vi "Micro-Epsilon ILD1420.vi"() -> (0 "DAQ Error":errorcluster)   [LabVIEW 2016]
uses:
  Globals/Meas_global.vi
panel:
  out "Waveform Graph":cluster{"y":dbl, dbl, "d (mm)":dbl[]}(graph)
  in  "Reconfigure settings":bool
  in  "Data rate (kHz)":string(combo)="0.25"
  in  "Measuring range (mm)":u8(ring)=4 items=["10", "25", "50", "100", "200"]
  in  "Auto laser off":bool=TRUE
  # "(set true if changing data rate)"
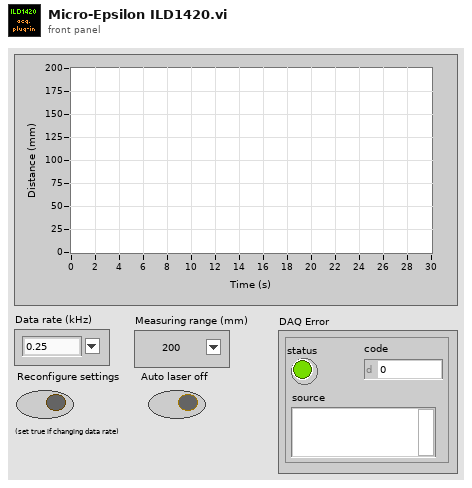
[diagram p1: front panel]
types:
  T1 = typedef "Analysis_info_cluster.ctl" = cluster{"Colour":u32, "Inst type":T2, "Inst name":string, "Symbol":string, "Code name":string, "Extra Info":string, "Inst Array":T3, "Extra Titles":string[], "Extra Values":string[], "U":dbl, "u^2":dbl, "u^3":dbl, "u^4":dbl, "Skew_u":dbl, "Kurt_u":dbl, "Sd Error in Mean":dbl, "% u'/U":dbl, "X":dbl, "Y":dbl, "Z":dbl, "Timescale integral Estimate":dbl, "Sd Error in Variance":dbl, "Calib File":path, "Calib Constants":dbl[], "Output Position":bool, "Full Stats":bool, "Av Sampling Rate":dbl, "Av No of Samples":dbl, "Total Meas Time (s)":dbl, "ADAM Ch Name":string, "Max value":dbl, "Min value":dbl}
  T2 = typedef "Inst_type.ctl" = enum16{"Propeller anemometer", "Raw voltage", "Pressure Transducer", "Pitot-static tube", "Preston tube", "Hot wire", "Cross wire 1", "Cross wire 2", "Generic Linear", "Generic Polynomial", "Generic BackPoly", "Fast FID", "Thermocouple", "Cold wire", "Pulsed Wire", "LDA Vel", "LDA Tran time", "LDA Arr time", "Microphone"}
  T3 = typedef "Instrument_Array.ctl" = enum16{"PWA", "LDA", "Analogue"}
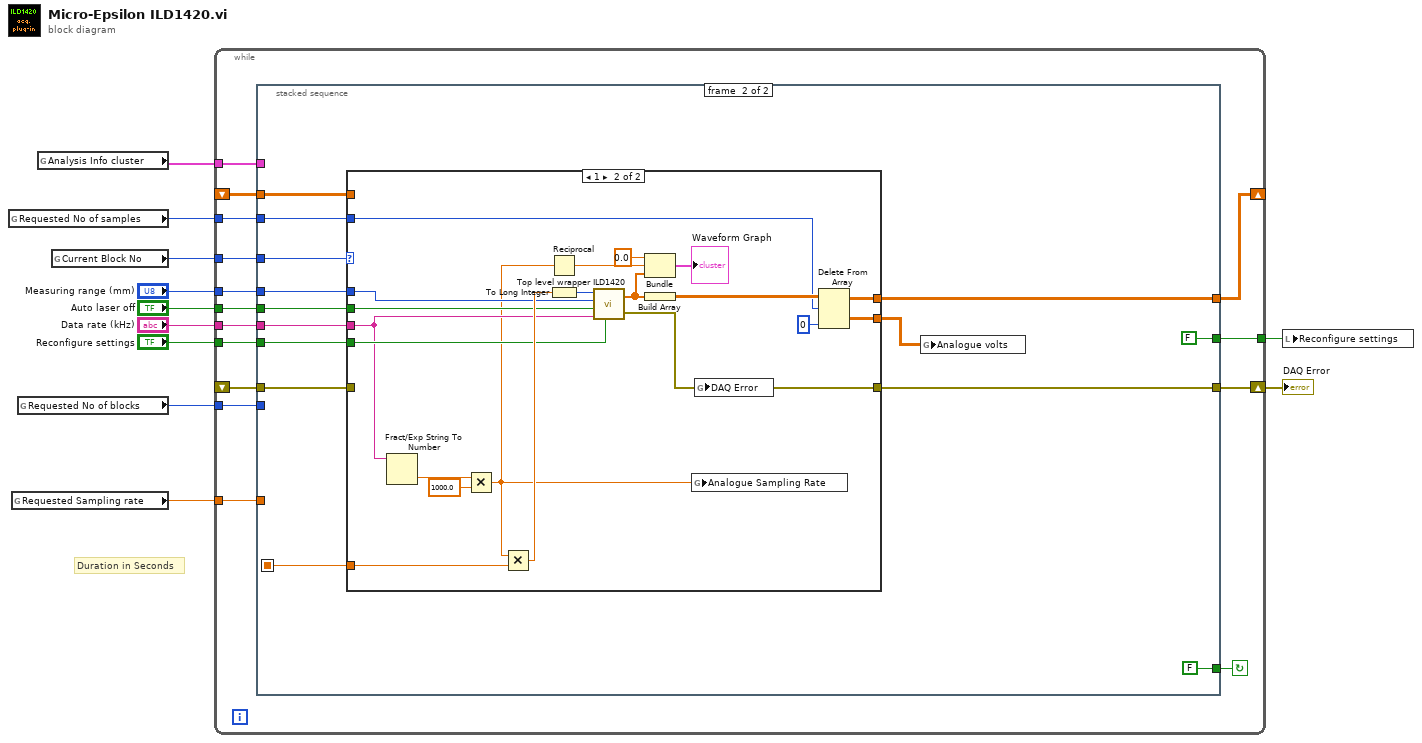
[diagram p0: block diagram]
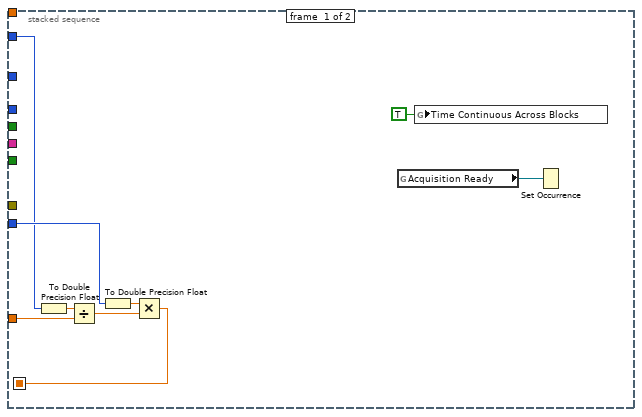
[diagram p2: hidden frame]
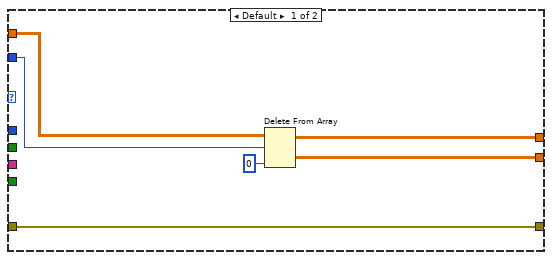
[diagram p3: hidden frame]
diagram:
  # "Duration in Seconds"
  n1 = global read "Meas_global.vi" "Requested No of samples"() -> (w11:i32)
  n2 = global read "Meas_global.vi" "Requested Sampling rate"() -> (w10:dbl)
  n3 = global read "Meas_global.vi" "Requested No of blocks"() -> (w7:i32)
  n4 = global read "Meas_global.vi" "Analysis Info cluster"() -> (w8:T1[])
  n5 = global read "Meas_global.vi" "Current Block No"() -> (w9:i32)
  n6 = while {
    tunnel: w11 -> [w26]
    tunnel: w10 -> [w25]
    tunnel: w9 -> [w24]
    tunnel: w8 -> [w23]
    tunnel: w7 -> [w22]
    tunnel: "Measuring range (mm)" -> [w20]
    tunnel: "Auto laser off" -> [w19]
    tunnel: "Data rate (kHz)" -> [w18]
    shift-right: [w14] -> _
    shift-left: _ -> [w12]
    tunnel: "Reconfigure settings" -> [w17]
    tunnel: [w16] -> w1
    shift-right: [w21] -> w6
    shift-left: _ -> [w13]
    stop <- w15 continue-if-true
    n7 = stacked-sequence {
      seq-local: [w32 _] -> [_ w49]
      tunnel: w26 -> [w31 w40]
      tunnel: w24 -> [_ w42]
      tunnel: w23 -> [_ _]
      tunnel: w25 -> [w35 _]
      tunnel: w22 -> [w33 _]
      tunnel: [_ w48] -> w21
      tunnel: w20 -> [_ w47]
      tunnel: w19 -> [_ w46]
      tunnel: w18 -> [_ w44]
      tunnel: w17 -> [_ w45]
      tunnel: [_ FALSE ("Reconfigure settings")] -> w16
      tunnel: [_ FALSE ("Reconfigure settings")] -> w15
      tunnel: [_ w39] -> w14
      tunnel: w13 -> [_ w38]
      tunnel: w12 -> [_ w37]
      frame #0 {
        n8 = To Double Precision Float(number=w31) -> (double precision float=w28:dbl)
        n9 = Divide(x=w28, y=w35) -> (x/y=w34:dbl)
        n10 = To Double Precision Float(number=w33) -> (double precision float=w27:dbl)
        n11 = Multiply(x=w27, y=w34) -> (x*y=w32:dbl)
        n12 = global read "Meas_global.vi" "Acquisition Ready"() -> (w29:refnum<k4>)
        n13 = global write "Meas_global.vi" "Time Continuous Across Blocks"(TRUE ("Time Continuous across Blocks")) -> ()
        n14 = Set Occurrence(w29) -> ()
      }
      frame #1 {
        n15 = case shown="1" w42 {
          tunnel: w49 -> [_ w75]
          tunnel: [w55 w73] -> w48
          tunnel: w47 -> [_ w71]
          tunnel: w46 -> [_ w70]
          tunnel: w45 -> [_ w69]
          tunnel: w44 -> [_ w68]
          tunnel: [w51 w58] -> w36
          tunnel: w40 -> [w52 w57]
          tunnel: [w50 w56] -> w39
          tunnel: w38 -> [w55 _]
          tunnel: w37 -> [w53 _]
          frame Default {
            n16 = Delete From Array(array=w53, length=w52, index (col)=0 ("disabled index (col)")) -> (deleted portion=w51:dbl[][], array with subset deleted=w50:dbl[][])  [unwired: 1 in]
          }
          frame 1 {
            n17 = Fract/Exp String To Number(string=w68) -> (number=w67:dbl)  [unwired: 3 in, 1 out]
            n18 = Multiply(x=w67, y=1000.0) -> (x*y=w63:dbl)
            n19 = Multiply(x=w63, y=w75) -> (x*y=w74:dbl)
            n20 = Reciprocal(x=w63) -> (1/x=w62:dbl)
            n21 = To Long Integer(number=w74) -> (32bit integer=w72:i32)
            n22 = call "Top level wrapper ILD1420.vi"("Reconfigure settings"=w69, "Data rate (kHz)"=w68, "Auto laser off"=w70, "Measuring range (mm)"=w71, "N samples"=w72) -> ("Error out"=w73:errorcluster, "d (mm)"=w65:dbl[])  [unwired: 1 in]
            n23 = Bundle("y"=0.0, w62, "d (mm)"=w65) -> (→"Waveform Graph":cluster{"y":dbl, dbl, "d (mm)":dbl[]})  [unwired: 1 in]
            n24 = Build Array(w65) -> (w59:dbl[][])
            n25 = global write "Meas_global.vi" "Analogue Sampling Rate"(w63) -> ()
            n26 = global write "Meas_global.vi" "DAQ Error"(w73) -> ()
            n27 = Delete From Array(array=w59, length=w57, index (col)=0 ("disabled index (col)")) -> (deleted portion=w58:dbl[][], array with subset deleted=w56:dbl[][])  [unwired: 1 in]
          }
        }
        n28 = global write "Meas_global.vi" "Analogue volts"(w36) -> ()
      }
    }
  }
  "DAQ Error" <- w6
  n29 = local write "Reconfigure settings"(w1) -> ()
